vi "Unit Test - Is CSM Modules.vi"() -> (3 "output cluster":cluster{T1[], T1[]})   [LabVIEW 2017, in "testcase-csmhelper.lvclass"]
uses:
  testcase-csmhelper.lvclass
  src/user.lib/_NEVSTOP/Communicable State Machine(CSM)/_csmHelper/Utility/CSM Module Type.ctl
  <vilib>/Utility/traverseref.llb/TRef TravTarget.ctl
  src/user.lib/_NEVSTOP/Communicable State Machine(CSM)/_csmHelper/Utility/CSM-Helper Utility.lvlib
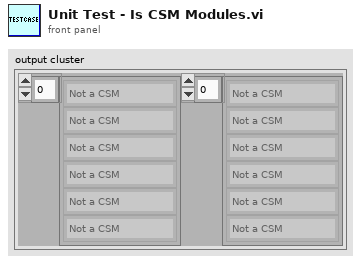
[diagram p1: front panel]
types:
  T1 = typedef "CSM-Helper Utility.lvlib/CSM Module Type.ctl" = enum16{"Not a CSM", "JKISM", "CSM"}
  T2 = typedef "TRef TravTarget.ctl" = enum16{"FP", "BD", "Other"}
  T3 = typedef "CSM-Helper Utility.lvlib/CSM Basic Refs.ctl" = cluster{"VI":refnum<vi>, "While Loop":refnum<vi>, "Case Structure":refnum<vi>, "Parse State Queue":refnum<vi>, "Event Structure":refnum<vi>, "Type":T1, "InLvlibp":bool}
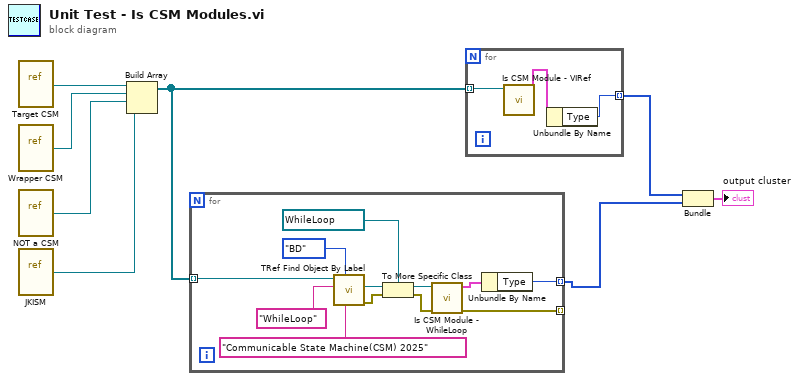
[diagram p0: block diagram]
diagram:
  n1 = vi-ref "Target CSM.vi"() -> (w6:refnum<vi>)
  n2 = vi-ref "Wrapper CSM.vi"() -> (w8:refnum<vi>)
  n3 = vi-ref "NOT a CSM.vi"() -> (w7:refnum<vi>)
  n4 = vi-ref "JKISM.vi"() -> (w4:refnum<vi>)
  n5 = Build Array(w6, w8, w7, w4) -> (w5:refnum<vi>[])
  n6 = for {
    tunnel: w5 -> [w20] mode=indexing
    tunnel: [w12] -> _ mode=indexing
    tunnel: [w9] -> w2 mode=indexing
    n7 = call <vilib>:"TRef Find Object By Label.vi"("Label"="Communicable State Machine(CSM) 2025", "Traverse Target"=TRef_TravTarget."BD", "Class Name"="WhileLoop", "VI Ref"=w20) -> ("error out"=w14:errorcluster, "Found Obj Ref"=w17:refnum<vi>)  [unwired: 4 in, 2 out]
    n8 = To More Specific Class(target class=refnum<vi> refnum ("WhileLoop in"), reference=w17, error in=w14) -> (specific class reference=w16:refnum<vi>, error out=w13:errorcluster)
    n9 = call "Is CSM Module - WhileLoop.vi"("error in (no error)"=w13, "WhileLoop in"=w16) -> ("error out"=w12:errorcluster, "CSM Basic Refs"=w10:T3)  [unwired: 6 in, 2 out]
    n10 = Unbundle By Name(w10) -> ("Type"=w9:T1)
  }
  n11 = for {
    tunnel: w5 -> [w23] mode=indexing
    tunnel: [w21] -> w3 mode=indexing
    n12 = call "Is CSM Module - VIRef.vi"("VIRef"=w23) -> ("CSM Basic Refs"=w22:T3)  [unwired: 7 in, 3 out]
    n13 = Unbundle By Name(w22) -> ("Type"=w21:T1)
  }
  n14 = Bundle(w3, w2) -> (→"output cluster":cluster{T1[], T1[]})  [unwired: 1 in]
